vi "Fs_to_FilterDelay.vi"(9 "Fs":dbl, 10 "DAQ Type":T1) -> (1 "Total Filter Delay (samples)":i32)   [LabVIEW 2016, in "Lockin.DAQ.lvclass"]
uses:
  Lockin.DAQ.lvclass
  Typedefs/DAQType-enum.ctl
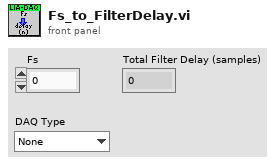
[diagram p1: front panel]
types:
  T1 = typedef "Lockin.DAQ.lvclass/DAQType-enum.ctl" = enum16{"None", "USB 4431", "PXI 446x"}
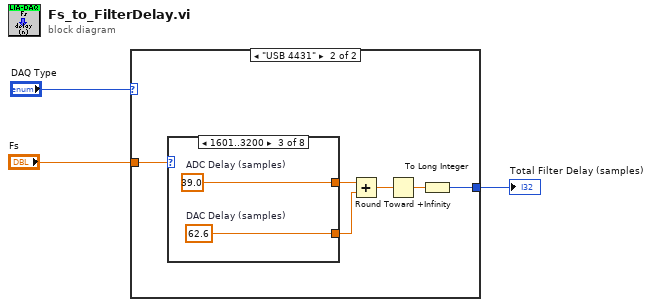
[diagram p0: block diagram]
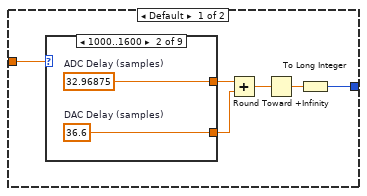
[diagram p2: hidden frame]
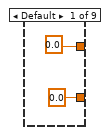
[diagram p3: hidden frame]
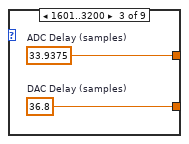
[diagram p4: hidden frame]
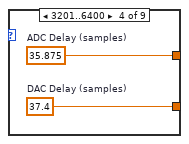
[diagram p5: hidden frame]
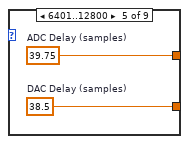
[diagram p6: hidden frame]
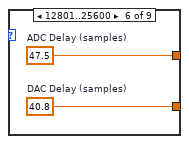
[diagram p7: hidden frame]
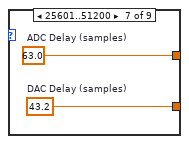
[diagram p8: hidden frame]
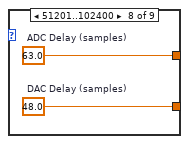
[diagram p9: hidden frame]
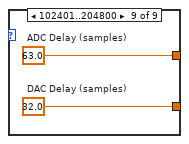
[diagram p10: hidden frame]
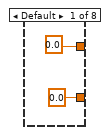
[diagram p11: hidden frame]
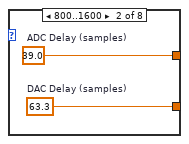
[diagram p12: hidden frame]
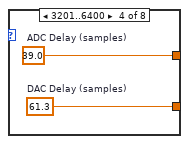
[diagram p13: hidden frame]
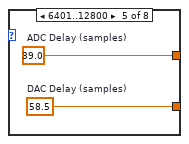
[diagram p14: hidden frame]
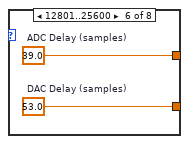
[diagram p15: hidden frame]
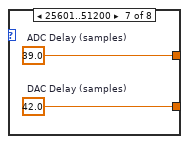
[diagram p16: hidden frame]
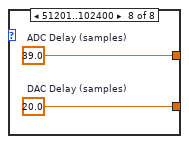
[diagram p17: hidden frame]
diagram:
  n1 = case shown="\"USB 4431\"" "DAQ Type" {
    tunnel: "Fs" -> [w5 w29]
    tunnel: [w4 w28] -> w1
    frame Default {
      n2 = case shown="1000..1600" w5 {
        tunnel: [0.0 ("ADC Delay (samples)") w13 w15 w17 w19 w21 w23 w25 w27] -> w6
        tunnel: [0.0 ("ADC Delay (samples)") w12 w14 w16 w18 w20 w22 w24 w26] -> w7
        frame Default {
        }
        frame 1000..1600 {
          w12 = 36.6  # DAC Delay (samples)
          w13 = 32.96875  # ADC Delay (samples)
        }
        frame 1601..3200 {
          w14 = 36.8  # DAC Delay (samples)
          w15 = 33.9375  # ADC Delay (samples)
        }
        frame 3201..6400 {
          w16 = 37.4  # DAC Delay (samples)
          w17 = 35.875  # ADC Delay (samples)
        }
        frame 6401..12800 {
          w18 = 38.5  # DAC Delay (samples)
          w19 = 39.75  # ADC Delay (samples)
        }
        frame 12801..25600 {
          w20 = 40.8  # DAC Delay (samples)
          w21 = 47.5  # ADC Delay (samples)
        }
        frame 25601..51200 {
          w23 = 63.0  # ADC Delay (samples)
          w22 = 43.2  # DAC Delay (samples)
        }
        frame 51201..102400 {
          w25 = 63.0  # ADC Delay (samples)
          w24 = 48.0  # DAC Delay (samples)
        }
        frame 102401..204800 {
          w27 = 63.0  # ADC Delay (samples)
          w26 = 32.0  # DAC Delay (samples)
        }
      }
      n3 = Add(x=w6, y=w7) -> (x+y=w8:dbl)
      n4 = Round Toward +Infinity(x=w8) -> (ceil(x): smallest int >= x=w9:dbl)
      n5 = To Long Integer(number=w9) -> (32bit integer=w4:i32)
    }
    frame "USB 4431" {
      n6 = case shown="1601..3200" w29 {
        tunnel: [0.0 ("ADC Delay (samples)") w37 w39 w41 w43 w45 w47 w49] -> w30
        tunnel: [0.0 ("ADC Delay (samples)") w36 w38 w40 w42 w44 w46 w48] -> w31
        frame Default {
        }
        frame 800..1600 {
          w36 = 63.3  # DAC Delay (samples)
          w37 = 39.0  # ADC Delay (samples)
        }
        frame 1601..3200 {
          w38 = 62.6  # DAC Delay (samples)
          w39 = 39.0  # ADC Delay (samples)
        }
        frame 3201..6400 {
          w40 = 61.3  # DAC Delay (samples)
          w41 = 39.0  # ADC Delay (samples)
        }
        frame 6401..12800 {
          w42 = 58.5  # DAC Delay (samples)
          w43 = 39.0  # ADC Delay (samples)
        }
        frame 12801..25600 {
          w44 = 53.0  # DAC Delay (samples)
          w45 = 39.0  # ADC Delay (samples)
        }
        frame 25601..51200 {
          w47 = 39.0  # ADC Delay (samples)
          w46 = 42.0  # DAC Delay (samples)
        }
        frame 51201..102400 {
          w49 = 39.0  # ADC Delay (samples)
          w48 = 20.0  # DAC Delay (samples)
        }
      }
      n7 = Add(x=w30, y=w31) -> (x+y=w32:dbl)
      n8 = Round Toward +Infinity(x=w32) -> (ceil(x): smallest int >= x=w33:dbl)
      n9 = To Long Integer(number=w33) -> (32bit integer=w28:i32)
    }
  }
  "Total Filter Delay (samples)" <- w1
